vi "initialize sys config device.vi"(8 "error in":errorcluster, 9 "login":cluster{"user name":string, "password":string}={"user name"="admin", "password"=""}, 10 "IP address (localhost)":string="localhost", 11 "controller in":refnum<class "Controller.lvclass">) -> (0 "error out":errorcluster, 3 "controller out":refnum<class "Controller.lvclass">)   [LabVIEW 2014, in "SMI.lvlib" / "SysCfg Device.lvclass"]
doc: "This VI initializes an NI System Configuration session when a valid NI Auth login is entered for the Real-Time target at the specified IP address."
uses:
  SysCfg Device.lvclass
  Controller/Controller.lvclass
  <vilib>/nisyscfg/Close (System).vi
  write password.vi
  write user name.vi
  write system session.vi
  <vilib>/nisyscfg/nisyscfg.lvlib
panel:
  # "NI Auth default settings are \nattempted automatically."
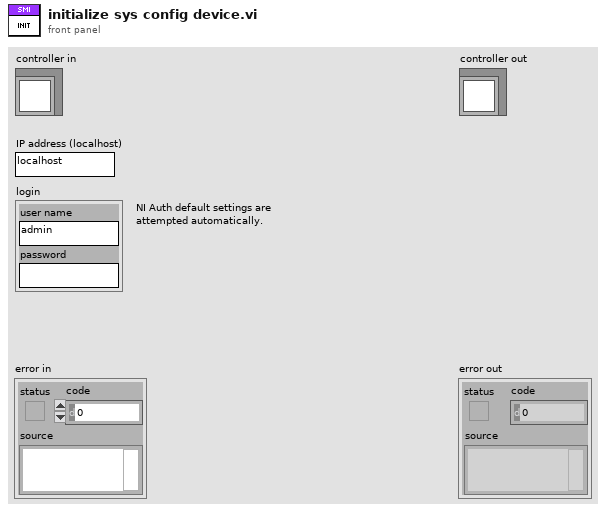
[diagram p1: front panel]
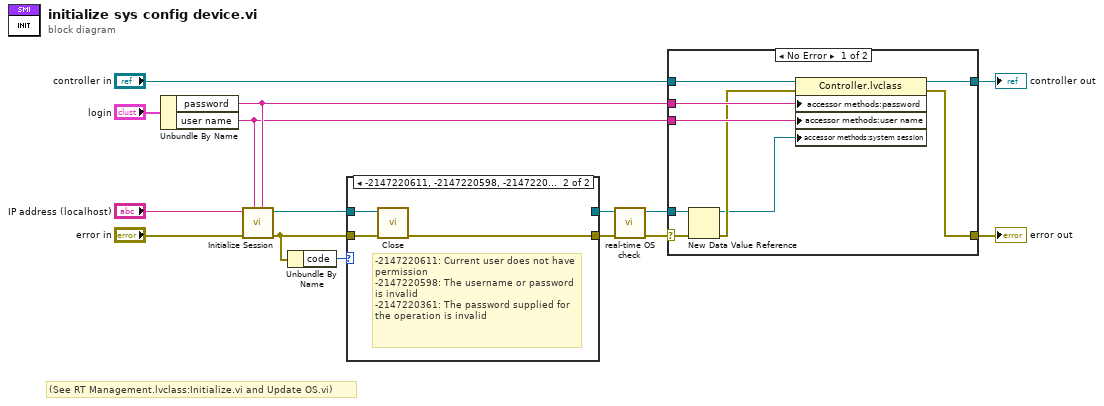
[diagram p0: block diagram]
diagram:
  # "(See RT Management.lvclass:Initialize.vi and Update OS.vi)"
  n1 = Unbundle By Name("login") -> ("password"=w13:string, "user name"=w12:string)
  n2 = call <vilib>:"Initialize Session.vi"("Password"=w13, "User Name"=w12, "error in (no error)"="error in", "Target (localhost)"="IP address (localhost)") -> ("error out"=w5:errorcluster, "Session out"=w4:refnum<k21>)  [unwired: 6 in]
  n3 = Unbundle By Name(w5) -> ("code"=w6:i32)
  n4 = case shown="-2147220611, -2147220598, -2147220361" w6 {
    tunnel: w4 -> [w17 w19]
    tunnel: w5 -> [w16 w20]
    tunnel: [w16 w18] -> w11
    tunnel: [w17 _] -> w10
    frame Default {
    }
    frame -2147220611, -2147220598, -2147220361 {
      # "-2147220611: Current user does not have permission\n-2147220598: The username or password is invalid \n-2147220361: The password supplied for the operation is invalid"
      n5 = call-poly <vilib>:"Close.vi"("error in (no error)"=w20, "Session in"=w19) -> ("error out"=w18:errorcluster)  [unwired: 9 in]
    }
  }
  n6 = call "real-time OS check.vi"("error in"=w11, "system session"=w10) -> ("error out"=w9:errorcluster, "system session out"=w3:refnum<k21>)  [unwired: 8 in]
  n7 = case shown="No Error" w9 {
    selector: w9 -> [w23 w31]
    tunnel: "controller in" -> [w29 w30]
    tunnel: [w28 w30] -> w15
    tunnel: w13 -> [w27 _]
    tunnel: w12 -> [w26 _]
    tunnel: [w25 w31] -> w8
    tunnel: w3 -> [w24 _]
    frame No Error {
      n8 = New Data Value Reference(data value=w24, error in=w23) -> (data value reference=w21:refnum<data-value>, error out=w22:errorcluster)
      n9 = property class="Controller.lvclass"(reference=w29, error in=w22, "accessor methods:password"=w27, "accessor methods:user name"=w26, "accessor methods:system session"=w21) -> (reference out=w28:refnum<class "Controller.lvclass">, error out=w25:errorcluster)
    }
    frame Error {
    }
  }
  "error out" <- w8
  "controller out" <- w15
